vi "diode characterization.vi"() -> ()   [LabVIEW 2018]
uses:
  <vilib>/Math Plots/3D Math Plots/3D Surface/3D Surface XCtrl/3D Surface.xctl
  <vilib>/DAQmx/write.llb/DAQmx Write (Analog Wfm 1Chan 1Samp).vi
  <vilib>/DAQmx/create/channels.llb/DAQmx Create Channel (AO-Voltage-Basic).vi
  <vilib>/Waveform/WDTOps.llb/WDT Get Waveform Subset DBL.vi
  <vilib>/DAQmx/miscellaneous.llb/DAQmx Fill In Error Info.vi
  <vilib>/Math Plots/3D Math Plots/3D Surface/3D Surface Datatype/Public/Plot Helper (Vector).vi
  <vilib>/Math Plots/3D Math Plots/3D Surface/3D Surface Datatype/3D Surface Datatype.lvclass
panel:
  in  "Voltage/Current In":tag="Dev2/ai0"
  in  "Voltage Out":tag="Dev2/ao0"
  out "Current":cluster{dbl[], dbl[]}(graph)
  out "Voltage":cluster{dbl[], dbl[]}(graph)
  in  "# of Iterations to Average":i32=1000
  out "Current Iteration #":i32
  out "3D Surface":refnum<class "3D Plot Datatype.lvclass">[](xcontrol)
  out "Power":cluster{dbl[], dbl[]}(graph)
  in  "dt":dbl max=1.0 step=0.01
  in  "Vmin":dbl
  in  "Vmax":dbl
  in  "Period":dbl=10.0 format="%.2g"
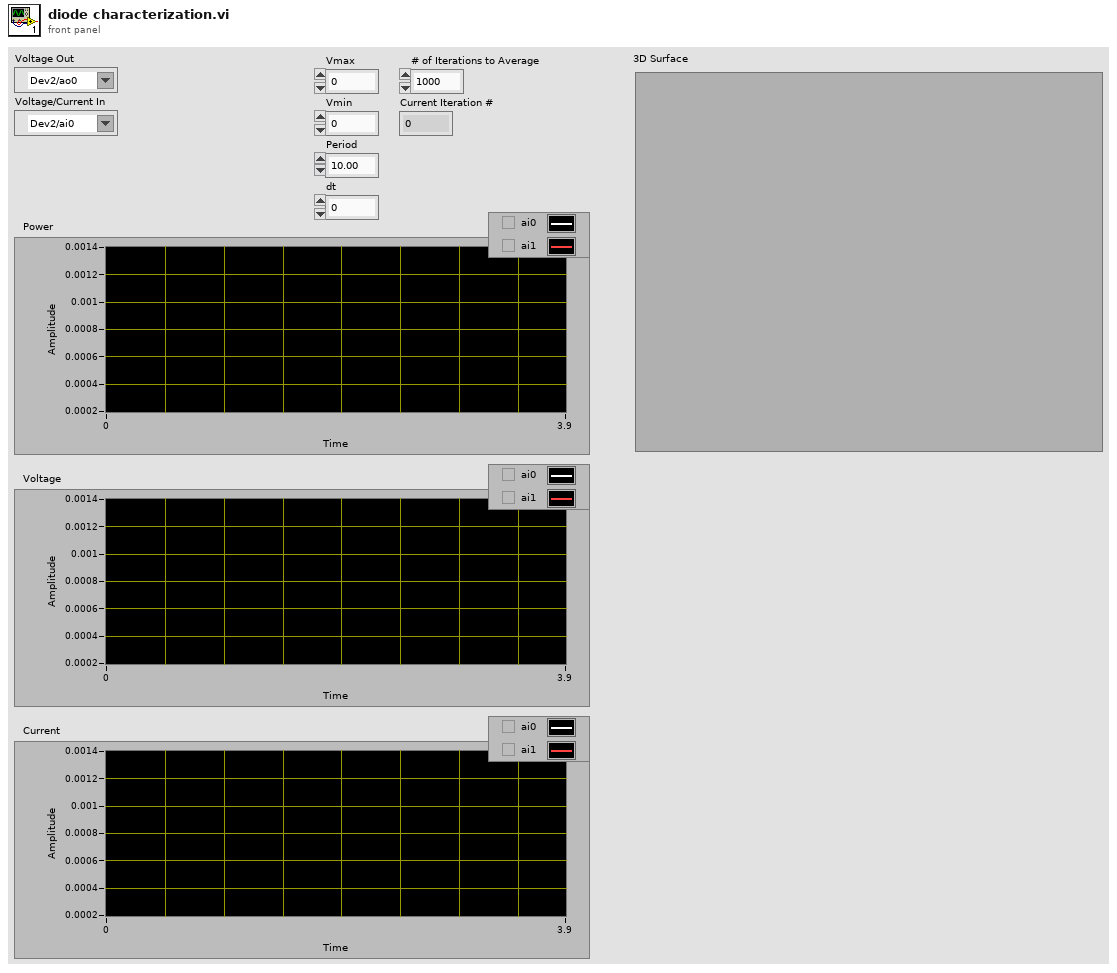
[diagram p1: front panel]
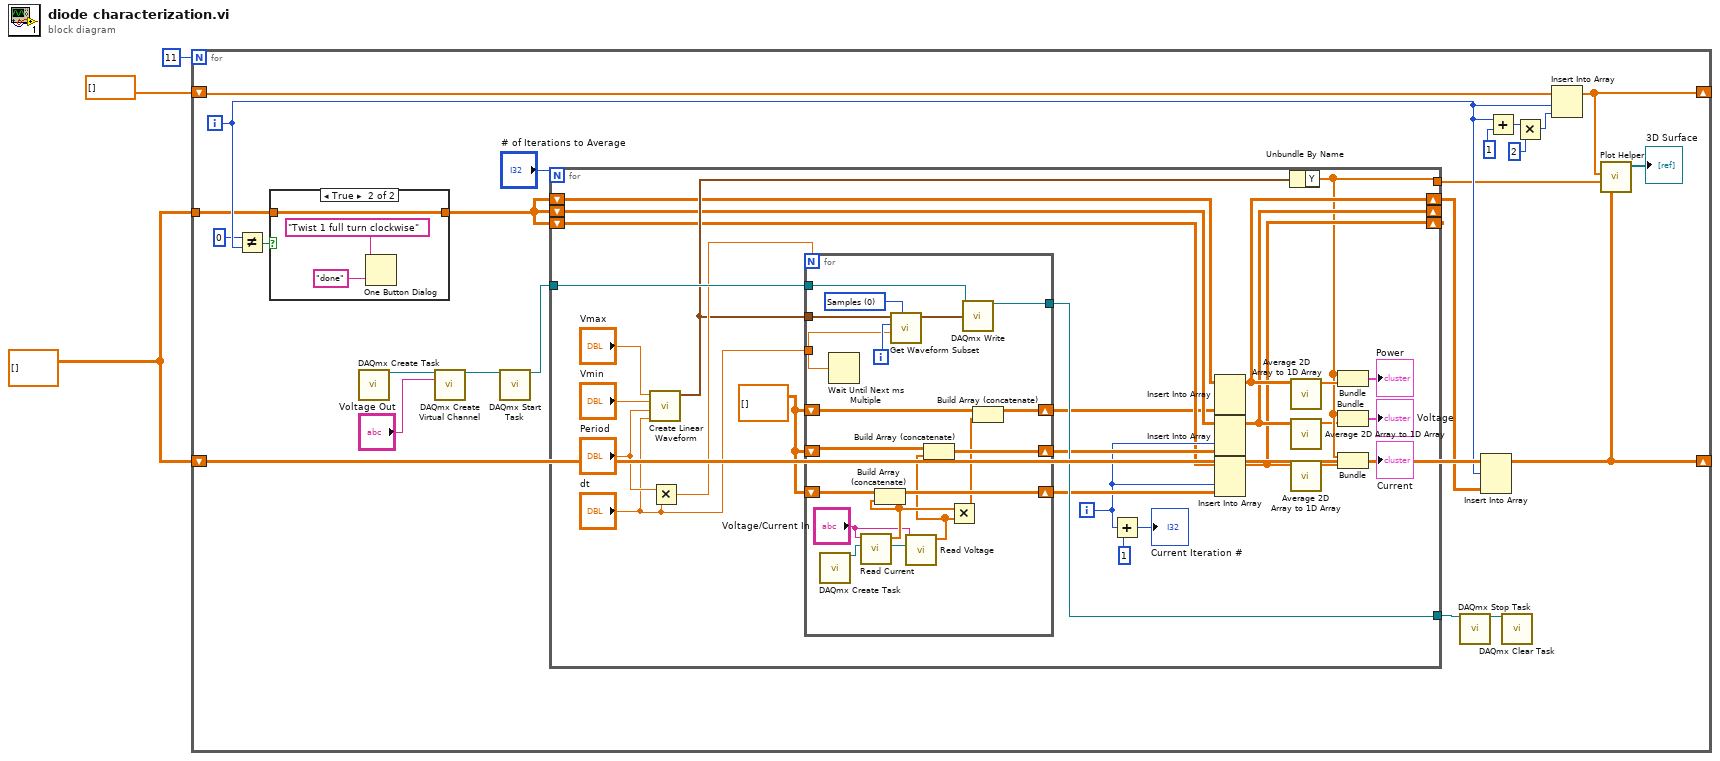
[diagram p0: block diagram]
diagram:
  w3 = dbl[][] []
  n1 = for {
    N: 11 -> [_]
    shift-right: [w18] -> _
    shift-left: w3 -> [w26]
    tunnel: w3 -> [w7]
    shift-right: [w19] -> _
    shift-left: dbl[] [] -> [w25]
    i -> [w17]
    n2 = Not Equal?(x=0, y=w17) -> (x != y?=w15:bool)
    n3 = case shown="True" w15 {
      tunnel: w7 -> [w74 w75]
      tunnel: [w74 w75] -> w5
      frame False {
      }
      frame True {
        n4 = One Button Dialog(message="Twist 1 full turn clockwise", button name ("OK")="done") -> ()  [unwired: 1 out]
      }
    }
    n5 = call <vilib>:"DAQmx Create Task.vi"() -> ("task out"=w12:refnum<k21>)  [unwired: 14 in, 1 out]
    n6 = call-poly <vilib>:"DAQmx Create Virtual Channel.vi"("task in"=w12, "physical channels"="Voltage Out") -> ("task out"=w11:refnum<k21>)  [unwired: 12 in, 1 out]
    n7 = call <vilib>:"DAQmx Start Task.vi"("task/channels in"=w11) -> ("task out"=w6:refnum<k21>)  [unwired: 13 in, 1 out]
    n8 = for {
      N: "# of Iterations to Average" -> [_]
      tunnel: w6 -> [w54]
      tunnel: [w53] -> w9
      shift-right: [w36] -> w4
      tunnel: [w29] -> w16
      shift-left: w5 -> [w40]
      shift-right: [w35] -> _
      shift-left: w5 -> [w39]
      shift-right: [w34] -> _
      shift-left: w5 -> [w38]
      i -> [w50]
      w41 = dbl[][] []
      n9 = call "Create Linear Waveform.vi"("dt"="dt", "Period"="Period", "Vmin"="Vmin", "Vmax"="Vmax") -> ("signal out"=w42:waveform(dbl))  [unwired: 7 in]
      n10 = Multiply(x="Period", y="dt") -> (x*y=w43:dbl)
      n11 = for {
        N: w43 -> [_]
        tunnel: w54 -> [w73]
        tunnel: [w72] -> w53
        tunnel: w42 -> [w70]
        tunnel: "dt" -> [w63]
        shift-right: [w65] -> w51
        shift-left: w41 -> [w66]
        shift-right: [w67] -> w52
        shift-left: w41 -> [w68]
        shift-right: [w61] -> w37
        shift-left: w41 -> [w62]
        i -> [w71]
        w64 = u16 0 items=["Samples", "Relative Time"] ("start/duration format")
        n12 = call <vilib>:"DAQmx Create Task.vi"() -> ("task out"=w59:refnum<k21>)  [unwired: 14 in, 1 out]
        n13 = Wait Until Next ms Multiple(millisecond multiple=w63) -> ()  [unwired: 1 out]
        n14 = call "Read Current.vi"("task in"=w59, "physical channels"="Voltage/Current In") -> ("task out"=w58:refnum<k21>, "data"=w57:dbl[])  [unwired: 8 in]
        n15 = Build Array (concatenate)(w68, w57) -> (w67:dbl[][])
        n16 = call-poly <vilib>:"Get Waveform Subset.vi"("start/duration format"=w64, "duration"=w63, "start samples/time"=w71, "waveform in"=w70) -> ("waveform out"=w69:waveform(dbl))  [unwired: 2 in, 3 out]
        n17 = call "Read Voltage.vi"("task in"=w58, "physical channels"="Voltage/Current In") -> ("data"=w56:dbl[])  [unwired: 8 in, 1 out]
        n18 = Build Array (concatenate)(w66, w56) -> (w65:dbl[][])
        n19 = Multiply(x=w57, y=w56) -> (x*y=w60:dbl[])
        n20 = call-poly <vilib>:"DAQmx Write.vi"("task/channels in"=w73, "data"=w69) -> ("task out"=w72:refnum<k21>)  [unwired: 11 in, 2 out]
        n21 = Build Array (concatenate)(w62, w60) -> (w61:dbl[][])
      }
      n22 = Add(x=w50, y=1) -> (x+y=→"Current Iteration #":i32)
      n23 = Insert Into Array(array=w40, new element=w37) -> (w36:dbl[][])  [unwired: 2 in]
      n24 = Insert Into Array(array=w39, index (col)=w50, new element=w51) -> (w35:dbl[][])  [unwired: 1 in]
      n25 = Insert Into Array(array=w38, index (col)=w50, new element=w52) -> (w34:dbl[][])  [unwired: 1 in]
      n26 = Unbundle By Name(w42) -> ("Y"=w29:dbl[])
      n27 = call "Average 2D Array to 1D Array.vi"("Array"=w36) -> ("Array 2"=w32:dbl[])  [unwired: 10 in]
      n28 = call "Average 2D Array to 1D Array.vi"("Array"=w35) -> ("Array 2"=w28:dbl[])  [unwired: 10 in]
      n29 = call "Average 2D Array to 1D Array.vi"("Array"=w34) -> ("Array 2"=w27:dbl[])  [unwired: 10 in]
      n30 = Bundle("Y"=w29, "Array 2"=w32) -> (→"Power":cluster{"Y":dbl[], "Array 2":dbl[]})  [unwired: 1 in]
      n31 = Bundle("Y"=w29, "Array 2"=w28) -> (→"Voltage":cluster{"Y":dbl[], "Array 2":dbl[]})  [unwired: 1 in]
      n32 = Bundle("Y"=w29, "Array 2"=w27) -> (→"Current":cluster{"Y":dbl[], "Array 2":dbl[]})  [unwired: 1 in]
    }
    n33 = call <vilib>:"DAQmx Stop Task.vi"("task/channels in"=w9) -> ("task out"=w10:refnum<k21>)  [unwired: 13 in, 1 out]
    n34 = Insert Into Array(array=w26, index (row)=w17, new element=w4) -> (w18:dbl[][])  [unwired: 1 in]
    n35 = Add(x=w17, y=1) -> (x+y=w24:i32)
    n36 = call <vilib>:"DAQmx Clear Task.vi"("task in"=w10) -> ()  [unwired: 14 in, 1 out]
    n37 = Multiply(x=w24, y=2) -> (x*y=w22:i32)
    n38 = Insert Into Array(array=w25, index=w17, new element=w22) -> (w19:dbl[])
    n39 = call-poly <vilib>:"Plot Helper.vi"("z matrix"=w18, "y vector"=w16, "x vector"=w19) -> ("3D Plot lvclass Array out"=→"3D Surface":refnum<class "3D Plot Datatype.lvclass">[])  [unwired: 3 in, 5 out]
  }
